vi "Get Server DLL Path.vi"() -> (0 "Server dll path":path)   [LabVIEW 2019, in "HVC9.lvlib" / "gprc-lvsupport.lvlib"]
uses:
  gprc-lvsupport.lvlib
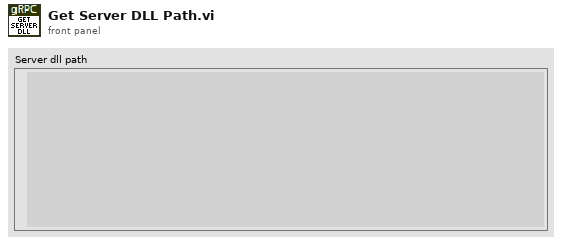
[diagram p1: front panel]
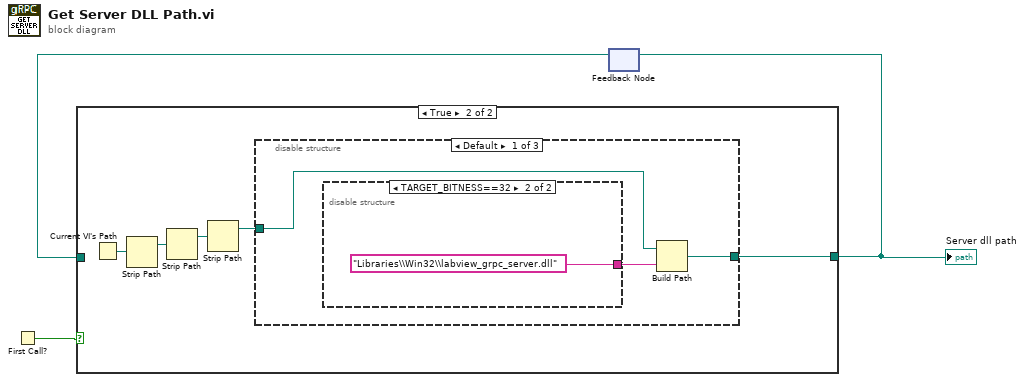
[diagram p0: block diagram]
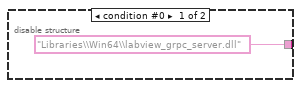
[diagram p3: hidden frame]
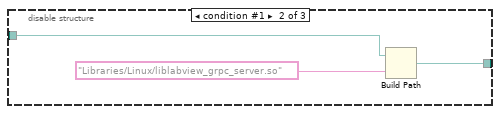
[diagram p4: hidden frame]
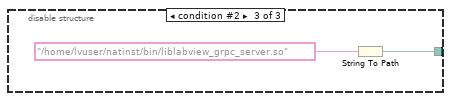
[diagram p5: hidden frame]
diagram:
  n1 = First Call?() -> (First Call?: T/F=w3:bool)
  n2 = feedback #1() -> (w1:path)  [unwired: 1 in]
  n3 = case shown="True" w3 {
    tunnel: [w4 w5] -> w2
    tunnel: w1 -> [w4 _]
    frame False {
    }
    frame True {
      n4 = Current VI's Path() -> (path=w8:path)
      n5 = Strip Path(path=w8) -> (stripped path=w9:path)  [unwired: 1 out]
      n6 = Strip Path(path=w9) -> (stripped path=w7:path)  [unwired: 1 out]
      n7 = Strip Path(path=w7) -> (stripped path=w6:path)  [unwired: 1 out]
      n8 = disable-structure shown="Default" {
        disable-tunnel: w6 -> [w11 w17 _]
        disable-tunnel: [w10 w16 w18] -> w5
        frame condition #0 (active) {
          n9 = disable-structure shown="TARGET_BITNESS==32" {
            disable-tunnel: ["Libraries\\Win64\\labview_grpc_server.dll" ("name or relative path") "Libraries\\Win32\\labview_grpc_server.dll" ("name or relative path")] -> w12
            frame condition #0 {
            }
            frame condition #1 (active) {
            }
          }
          n10 = Build Path(base path=w11, name or relative path=w12) -> (appended path=w10:path)
        }
        frame condition #1 {
          n11 = Build Path(base path=w17, name or relative path="Libraries/Linux/liblabview_grpc_server.so") -> (appended path=w16:path)
        }
        frame condition #2 {
          n12 = String To Path(string="/home/lvuser/natinst/bin/liblabview_grpc_server.so" ("name or relative path")) -> (path=w18:path)
        }
      }
    }
  }
  "Server dll path" <- w2
  n13 = feedback-in #1(w2) -> ()
